vi "Intruder_Final.vi"() -> ()   [LabVIEW 2020]
uses:
  <vilib>/Instr/_visa.llb/VISA Flush IO Buffer Mask.ctl
  <vilib>/ptbypt/NI_PtbyPt.lvlib
  <vilib>/httpClient/LabVIEWHTTPClient.lvlib
  <vilib>/DAQmx/create/channels.llb/DAQmx Create Channel (DI-Digital Input).vi
  <vilib>/Instr/_visa.llb/VISA Configure Serial Port (Instr).vi
  <vilib>/DAQmx/read.llb/DAQmx Read (Digital Bool 1Line 1Point).vi
  <vilib>/DAQmx/create/channels.llb/DAQmx Create Channel (DO-Digital Output).vi
  <vilib>/DAQmx/write.llb/DAQmx Write (Digital Bool 1Line 1Point).vi
  <vilib>/httpClient/PUTBuffer.vi
panel:
  out "Buzzer":bool
  in  "Buzzer Pin":tag
  out "Touch":bool
  out "PIR":bool
  in  "PIR":tag
  in  "Touch":tag
  out "Centimeters":i32
  out "Error Out":errorcluster
  in  "System Armed?":bool
  out "Boolean":bool
  out "Iteration":i32
  out "Present (s)":dbl
  out "Elapsed Time (s)":dbl
  in  "STOP":bool
  out "INTRUDER ALERT ALERT!":bool
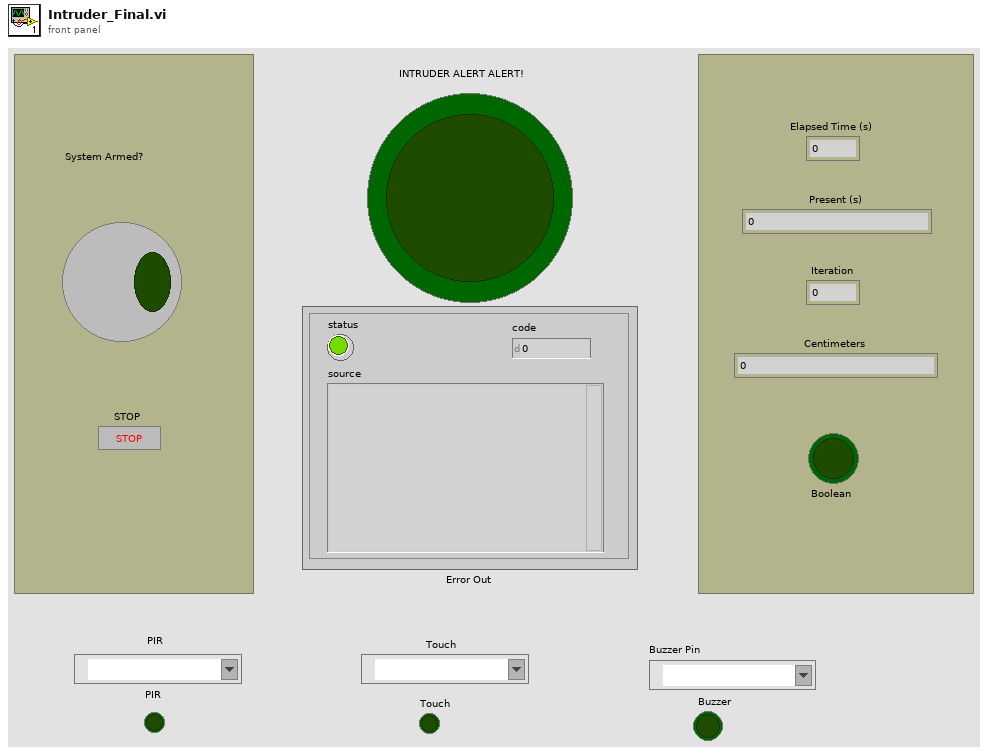
[diagram p1: front panel]
types:
  T1 = typedef "VISA Flush IO Buffer Mask.ctl" = u16
  T2 = typedef "LabVIEWHTTPClient.lvlib/ClientHandle.ctl" = refnum<k1>
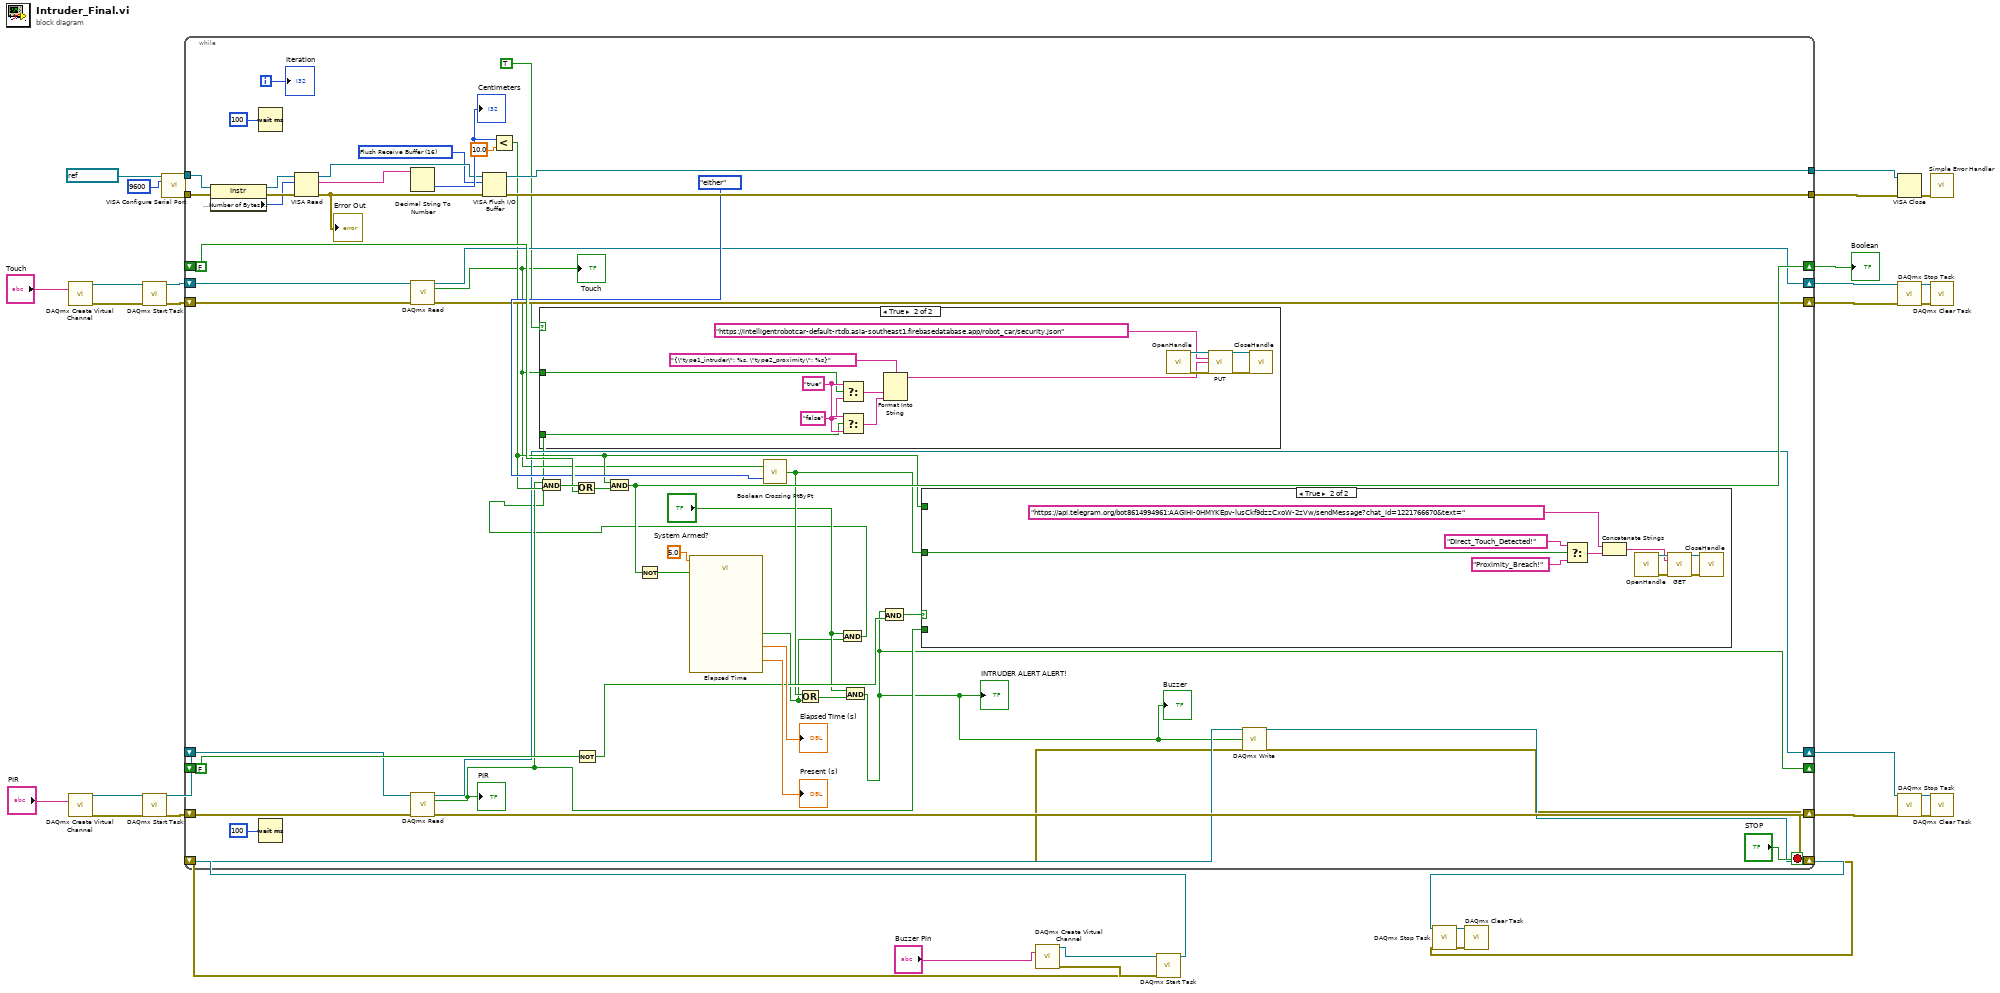
[diagram p0: block diagram]
diagram:
  n1 = call-poly <vilib>:"DAQmx Create Virtual Channel.vi"("lines"="Touch") -> ("task out"=w27:refnum<k21>, "error out"=w26:errorcluster)  [unwired: 13 in]
  n2 = call-poly <vilib>:"DAQmx Create Virtual Channel.vi"("lines"="PIR") -> ("task out"=w18:refnum<k21>, "error out"=w17:errorcluster)  [unwired: 13 in]
  n3 = call <vilib>:"DAQmx Start Task.vi"("task/channels in"=w27, "error in"=w26) -> ("task out"=w20:refnum<k21>, "error out"=w19:errorcluster)  [unwired: 12 in]
  n4 = call <vilib>:"DAQmx Start Task.vi"("task/channels in"=w18, "error in"=w17) -> ("task out"=w15:refnum<k21>, "error out"=w14:errorcluster)  [unwired: 12 in]
  n5 = call-poly "VISA Configure Serial Port"("VISA resource name"=refnum<visa-resource-name> "COM25", "baud rate (9600)"=u32 9600) -> ("VISA resource name out"=w32:refnum<visa-resource-name>, "error out"=w31:errorcluster)  [unwired: 12 in]
  n6 = call-poly <vilib>:"DAQmx Create Virtual Channel.vi"("lines"="Buzzer Pin") -> ("task out"=w8:refnum<k21>, "error out"=w7:errorcluster)  [unwired: 13 in]
  n7 = call <vilib>:"DAQmx Start Task.vi"("task/channels in"=w8, "error in"=w7) -> ("task out"=w6:refnum<k21>, "error out"=w5:errorcluster)  [unwired: 12 in]
  n8 = while {
    shift-right: [w84] -> w36
    shift-left: FALSE -> [w83]
    shift-right: [w40] -> _
    shift-left: FALSE -> [w76]
    tunnel: w32 -> [w72]
    tunnel: w31 -> [w71]
    tunnel: [w67] -> w29
    tunnel: [w66] -> w28
    shift-right: [w59] -> w22
    shift-left: w20 -> [w57]
    shift-right: [w58] -> w21
    shift-left: w19 -> [w56]
    shift-right: [w50] -> w11
    shift-left: w15 -> [w52]
    shift-right: [w49] -> w10
    shift-left: w14 -> [w51]
    shift-right: [w39] -> w2
    shift-left: w6 -> [w42]
    shift-right: [w38] -> w1
    shift-left: w5 -> [w41]
    i -> [w79]
    stop <- "STOP" stop-if-true
    w63 = T1 16 items=["Flush Receive Buffer"=16, "Write Transmit Buffer to Device"=32, "Flush Receive Buffer (No I/O)"=64, "Flush Transmit Buffer"=128] ("Mask")
    n9 = property class="Instr"(reference=w72, error in=w71) -> (reference out=w70:refnum<visa-resource-name>, error out=w69:errorcluster, "Serial Settings:Number of Bytes at Serial Port"=w68:u32)
    n10 = Wait (ms)(milliseconds to wait=u32 100) -> ()  [unwired: 1 out]
    n11 = Wait (ms)(milliseconds to wait=u32 100) -> ()  [unwired: 1 out]
    n12 = VISA Read(VISA resource name=w70, byte count=w68, error in (no error)=w69) -> (VISA resource name out=w65:refnum<visa-resource-name>, read buffer=w73:string, error out=w64:errorcluster)  [unwired: 1 out]
    "Error Out" <- w64
    n13 = Decimal String To Number(string=w73) -> (number=w74:i32)  [unwired: 2 in, 1 out]
    "Centimeters" <- w74
    n14 = call-poly <vilib>:"DAQmx Read.vi"("task/channels in"=w57, "error in"=w56) -> ("task out"=w59:refnum<k21>, "data"=w47:bool, "error out"=w58:errorcluster)  [unwired: 11 in]
    "Touch" <- w47
    n15 = call-poly <vilib>:"DAQmx Read.vi"("task/channels in"=w52, "error in"=w51) -> ("task out"=w50:refnum<k21>, "data"=w46:bool, "error out"=w49:errorcluster)  [unwired: 11 in]
    "PIR" <- w46
    n16 = VISA Flush I/O Buffer(VISA resource name=w65, mask (16)=w63, error in (no error)=w64) -> (VISA resource name out=w67:refnum<visa-resource-name>, error out=w66:errorcluster)
    n17 = Less?(x=w74, y=10.0) -> (x < y?=w53:bool)
    n18 = And(x=w46, y=w53) -> (x .and. y?=w85:bool)
    n19 = Or(x=w85, y=w83) -> (x .or. y?=w87:bool)
    n20 = Not(x=w76) -> (.not. x?=w75:bool)
    n21 = And(x=w53, y=w87) -> (x .and. y?=w84:bool)
    n22 = Not(x=w84) -> (.not. x?=w78:bool)
    n23 = call "Elapsed Time"("Time Target (s)"=5.0, "Reset"=w78) -> ("Present (s)"=→"Present (s)":dbl, "Elapsed Time (s)"=→"Elapsed Time (s)":dbl, "Time has Elapsed"=w44:bool)  [unwired: 10 in, 5 out]
    n24 = call <vilib>:"Boolean Crossing PtByPt.vi"("direction"=enum16{"either", "false-true", "true-false"}."either", "input"=w47) -> ("crossing"=w54:bool)  [unwired: 1 in]
    n25 = Or(x=w54, y=w44) -> (x .or. y?=w77:bool)
    n26 = And(x="System Armed?", y=w44) -> (x .and. y?=w43:bool)
    n27 = case shown="True" TRUE {
      tunnel: w47 -> [_ w90]
      tunnel: w43 -> [_ w89]
      frame False {
      }
      frame True {
        w95 = "false"
        w96 = "true"
        n28 = Select(t=w96, s=w90, f=w95) -> (s? t:f=w93:string)
        n29 = Select(t=w96, s=w89, f=w95) -> (s? t:f=w92:string)
        n30 = Format Into String(format string="{\"type1_intruder\": %s, \"type2_proximity\": %s}", w93, w92) -> (resulting string=w91:string)  [unwired: 2 in, 1 out]
        n31 = call <vilib>:"OpenHandle.vi"() -> ("client handle out"=w100:T2, "error out"=w101:errorcluster)  [unwired: 14 in]
        n32 = call-poly <vilib>:"PUT.vi"("client handle"=w100, "url"="https://intelligentrobotcar-default-rtdb.asia-southeast1.firebasedatabase.app/robot_car/security.json", "buffer"=w91, "error in (no error)"=w101) -> ("client handle out"=w98:T2, "error out"=w99:errorcluster)  [unwired: 8 in, 2 out]
        n33 = call <vilib>:"CloseHandle.vi"("client handle"=w98, "error in (no error)"=w99) -> ()  [unwired: 13 in, 1 out]
      }
    }
    n34 = And(x="System Armed?", y=w77) -> (x .and. y?=w40:bool)
    "INTRUDER ALERT ALERT!" <- w40
    "Buzzer" <- w40
    n35 = And(x=w40, y=w75) -> (x .and. y?=w55:bool)
    n36 = case shown="True" w55 {
      tunnel: w46 -> [_ _]
      tunnel: w54 -> [_ w102]
      tunnel: w53 -> [_ _]
      frame False {
      }
      frame True {
        n37 = Select(t="Direct_Touch_Detected!", s=w102, f="Proximity_Breach!") -> (s? t:f=w106:string)
        n38 = Concatenate Strings("https://api.telegram.org/bot8614994961:AAGiHI-0HMYKEpv-lusCkf9dzzCxoW-2zVw/sendMessage?chat_id=1221766670&text=", w106) -> (w103:string)
        n39 = call <vilib>:"OpenHandle.vi"() -> ("client handle out"=w111:T2, "error out"=w110:errorcluster)  [unwired: 14 in]
        n40 = call <vilib>:"GET.vi"("client handle"=w111, "url"=w103, "error in (no error)"=w110) -> ("client handle out"=w109:T2, "error out"=w108:errorcluster)  [unwired: 9 in, 2 out]
        n41 = call <vilib>:"CloseHandle.vi"("client handle"=w109, "error in (no error)"=w108) -> ()  [unwired: 13 in, 1 out]
      }
    }
    n42 = call-poly <vilib>:"DAQmx Write.vi"("task/channels in"=w42, "data"=w40, "error in"=w41) -> ("task out"=w39:refnum<k21>, "error out"=w38:errorcluster)  [unwired: 10 in, 1 out]
    "Iteration" <- w79
  }
  "Boolean" <- w36
  n43 = call <vilib>:"DAQmx Stop Task.vi"("task/channels in"=w2, "error in"=w1) -> ("task out"=w4:refnum<k21>, "error out"=w3:errorcluster)  [unwired: 12 in]
  n44 = call <vilib>:"DAQmx Clear Task.vi"("task in"=w4, "error in"=w3) -> ()  [unwired: 13 in, 1 out]
  n45 = VISA Close(VISA resource name=w29, error in (no error)=w28) -> (error out=w30:errorcluster)
  n46 = call <vilib>:"DAQmx Stop Task.vi"("task/channels in"=w22, "error in"=w21) -> ("task out"=w24:refnum<k21>, "error out"=w23:errorcluster)  [unwired: 12 in]
  n47 = call <vilib>:"DAQmx Stop Task.vi"("task/channels in"=w11, "error in"=w10) -> ("task out"=w13:refnum<k21>, "error out"=w12:errorcluster)  [unwired: 12 in]
  n48 = call <vilib>:"Simple Error Handler.vi"("error in (no error)"=w30) -> ()  [unwired: 4 in, 5 out]
  n49 = call <vilib>:"DAQmx Clear Task.vi"("task in"=w24, "error in"=w23) -> ()  [unwired: 13 in, 1 out]
  n50 = call <vilib>:"DAQmx Clear Task.vi"("task in"=w13, "error in"=w12) -> ()  [unwired: 13 in, 1 out]
